vi "block_for_change.vi"(8 "error in (no error)":errorcluster, 9 "event_registration":refnum<event-registration>, 11 "timeout_ms":i32=1000) -> (0 "error out":errorcluster, 2 "data":variant, 3 "transition":bool)   [LabVIEW 2015, in "lv-recipe-machine.lvlib"]
uses:
  lv-recipe-machine.lvlib
  public/_controls/change.ctl
  public/_controls/transition.ctl
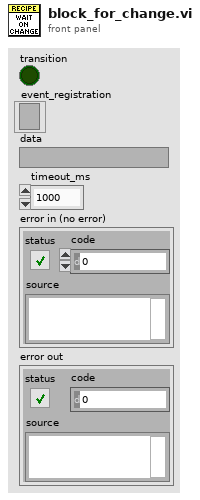
[diagram p1: front panel]
types:
  T1 = typedef "lv-recipe-machine.lvlib/transition.ctl" = cluster{"next_step":string, "next_index":i32, "data":variant, "error":errorcluster}
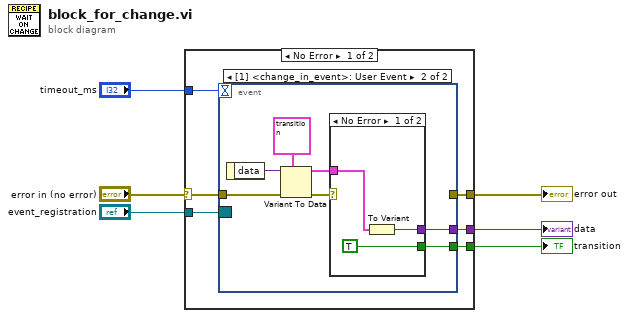
[diagram p0: block diagram]
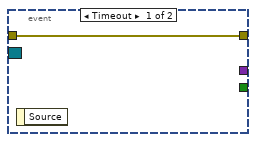
[diagram p2: hidden frame]
diagram:
  n1 = case shown="No Error" "error in (no error)" {
    selector: "error in (no error)" -> [w10 w24]
    tunnel: "timeout_ms" -> [w12 _]
    tunnel: "event_registration" -> [w11 _]
    tunnel: [w9 w24] -> w3
    tunnel: [w8 _] -> w2
    tunnel: [w7 _] -> w1
    frame No Error {
      n2 = event shown="[1] <change_in_event>: User Event" {
        selector: w11 -> [_ _]
        dyn-events: _ -> [_ _]
        timeout: w12 -> [_ _]
        tunnel: w10 -> [w13 w19]
        tunnel: [w13 _] -> w9
        tunnel: [_ w15] -> w8
        tunnel: [_ w14] -> w7
        event Timeout {
          n3 = event-data() -> ()  [unwired: 1 in, 1 out]
        }
        event User Event {
          n4 = event-data() -> ("data"=w20:variant)  [unwired: 1 in]
          n5 = Variant To Data(error in=w19, type=T1 {"next_step"="", "next_index"=-1, "data"=variant, "error"={"status"=FALSE, "code"=0, "source"=""}} ("transition"), Variant=w20) -> (data=w17:T1, error out=w16:errorcluster)
          n6 = case shown="No Error" w16 {
            tunnel: w17 -> [w22 _]
            tunnel: [w23 _] -> w15
            tunnel: [TRUE _] -> w14
            frame No Error {
              n7 = To Variant(anything=w22) -> (Variant=w23:variant)
            }
            frame Error {
            }
          }
        }
      }
    }
    frame Error {
    }
  }
  "error out" <- w3
  "transition" <- w1
  "data" <- w2
